vi "UI.vi"() -> ()   [LabVIEW 2016, in "余氯.lvlib"]
uses:
  PLC/PLC.lvlib
  <vilib>/ptbypt/NI_PtbyPt.lvlib
panel:
  in  "测试时间（s）":dbl=60.0
  in  "周期间隔（H）":dbl=4.0
  in  "修正系数":dbl=1.0
  in  "b":dbl=-0.5
  in  "K":dbl=0.000305213
  in  "AD通道":enum16{"AD0", "AD1", "AD2", "AD3", "AD4", "AD5"}(ring)=enum."AD2"
  out "余氯":dbl format="%#.2f"
  # "mg/L"
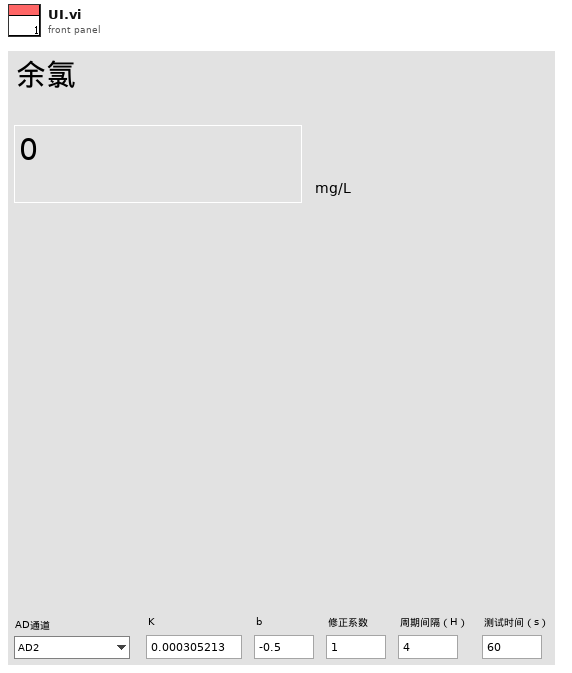
[diagram p1: front panel]
types:
  T1 = cluster{"AD通道":enum16{"AD0", "AD1", "AD2", "AD3", "AD4", "AD5"}, "K":dbl, "b":dbl, "修正系数":dbl, "周期间隔（H）":dbl, "测试时间（s）":dbl}
  T2 = enum16{"空闲", "润洗", "采样", "沉淀", "配水", "反冲洗", "储水", "结束"}
  T3 = typedef "流量计字段定义.ctl" = cluster{"时间":timestamp, "测量模式":string, "数据类型":string, "检测值":sgl, "单位":string, "数据标识":string, "因子编码":string}
  T4 = typedef "LVDateTimeRec.ctl" = cluster{"秒数的小数部分":dbl, "秒":i32, "分":i32, "时":i32, "日":i32, "月":i32, "年":i32, "天数（周）":i32, "天数（年）":i32, "DST":i32}
  T5 = cluster{"AD通道":enum16{"AD0", "AD1", "AD2", "AD3", "AD4", "AD5"}, "K":dbl, "b":dbl, "修正系数":dbl, "数据保存间隔":i32, "测试时间（s）":dbl}
  T6 = cluster{"AD0":i16, "AD1":i16, "AD2":i16, "AD3":i16, "AD4":i16, "AD5":i16}
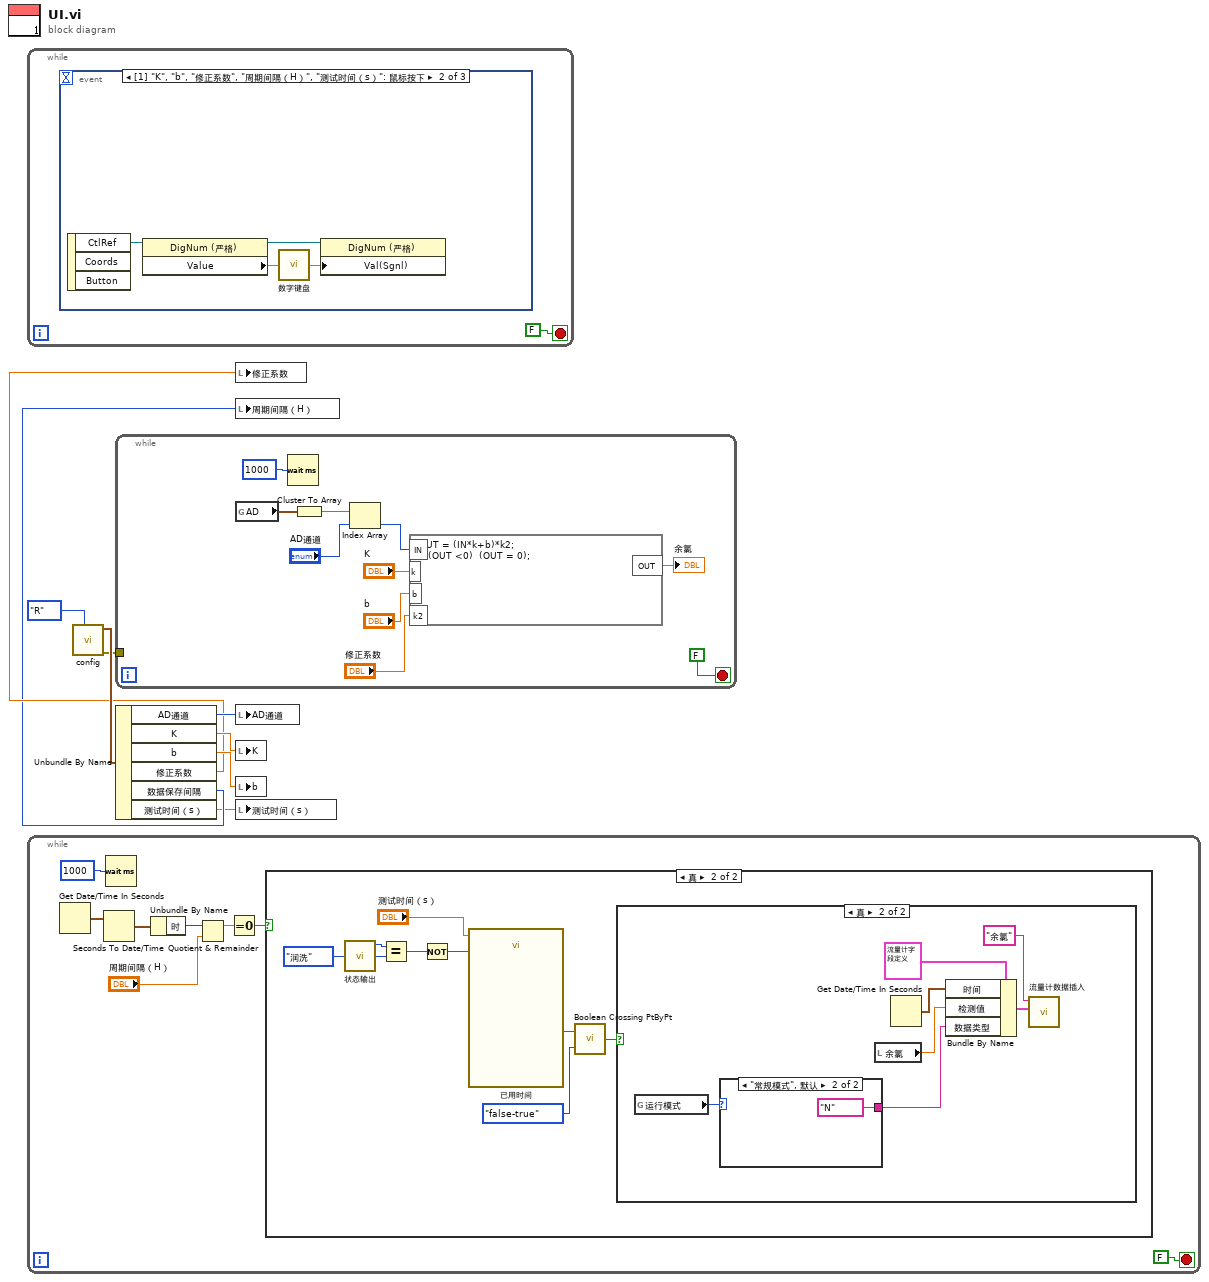
[diagram p0: block diagram]
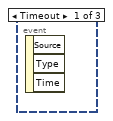
[diagram p2: hidden frame]
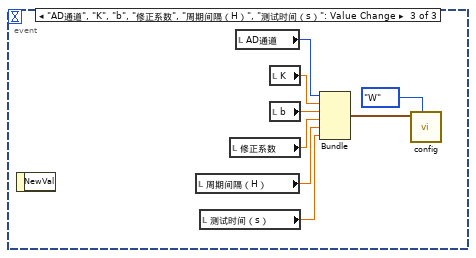
[diagram p3: hidden frame]
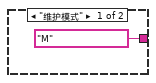
[diagram p6: hidden frame]
diagram:
  n1 = while {
    stop <- FALSE stop-if-true
    n2 = event shown="[1] \"K\", \"b\", \"修正系数\", \"周期间隔（H）\", \"测试时间（s）\": 鼠标按下" {
      selector: _ -> [_ _ _]
      dyn-events: _ -> [_ _ _]
      timeout: _ -> [_ _ _]
      event Timeout {
        n3 = event-data() -> ()  [unwired: 1 in, 3 out]
      }
      event "K", "b", "修正系数", "周期间隔（H）", "测试时间（s）": Mouse Down {
        n4 = event-data() -> ("CtlRef"=w14:refnum<vi>)  [unwired: 1 in, 2 out]
        n5 = property class="DigNum (严格)"(reference=w14) -> (reference out=w12:refnum<vi>, "Value"=w13:dbl)  [unwired: 1 in, 1 out]
        n6 = call "数字键盘.vi"("OldNumber"=w13) -> ("NewNumber"=w11:sgl)
        n7 = property class="DigNum (严格)"(reference=w12, "Val(Sgnl)"=w11) -> ()  [unwired: 1 in, 2 out]
      }
      event "AD通道", "K", "b", "修正系数", "周期间隔（H）", "测试时间（s）": Value Change {
        n8 = event-data() -> ()  [unwired: 1 in, 1 out]
        n9 = local read "周期间隔（H）"() -> (w16:dbl)
        n10 = local read "测试时间（s）"() -> (w15:dbl)
        n11 = local read "修正系数"() -> (w18:dbl)
        n12 = local read "AD通道"() -> (w21:enum16{"AD0", "AD1", "AD2", "AD3", "AD4", "AD5"})
        n13 = local read "K"() -> (w20:dbl)
        n14 = local read "b"() -> (w19:dbl)
        n15 = Bundle("AD通道"=w21, "K"=w20, "b"=w19, "修正系数"=w18, "周期间隔（H）"=w16, "测试时间（s）"=w15) -> (w17:T1)  [unwired: 1 in]
        n16 = call "config.vi"("FUN"=enum16{"R", "W"}."W", "配置输入"=w17) -> ()  [unwired: 8 in, 2 out]
      }
    }
  }
  n17 = while {
    stop <- FALSE stop-if-true
    n18 = Get Date/Time In Seconds() -> (seconds since 1Jan1904=w28:timestamp)
    n19 = Seconds To Date/Time(time stamp (now)=w28) -> (date time rec=w27:T4)  [unwired: 1 in]
    n20 = Wait (ms)(milliseconds to wait=u32 1000 ("等待时间（毫秒）")) -> ()  [unwired: 1 out]
    n21 = Unbundle By Name(w27) -> ("时"=w26:i32)
    n22 = Quotient & Remainder(x=w26, y="周期间隔（H）") -> (x-y*floor(x/y)=w24:dbl)  [unwired: 1 out]
    n23 = Equal To 0?(x=w24) -> (x = 0?=w23:bool)
    n24 = case shown="真" w23 {
      frame False {
      }
      frame True {
        n25 = call "状态输出.vi"() -> ("采配水流程"=w38:T2)  [unwired: 11 in]
        n26 = Equal?(x=w38, y=T2."润洗") -> (x = y?=w33:bool)
        n27 = Not(x=w33) -> (.not. x?=w32:bool)
        n28 = call "已用时间"("Time Target (s)"="测试时间（s）", "Reset"=w32) -> ("Time has Elapsed"=w31:bool)  [unwired: 10 in, 7 out]
        n29 = call <vilib>:"Boolean Crossing PtByPt.vi"("direction"=enum16{"either", "false-true", "true-false"}."false-true", "input"=w31) -> ("crossing"=w36:bool)  [unwired: 1 in]
        n30 = case shown="真" w36 {
          frame False {
          }
          frame True {
            n31 = global read "系统设置全局变量.vi" "运行模式"() -> (w40:enum16{"维护模式", "常规模式", "应急模式", "质控模式"})
            n32 = case shown="\"常规模式\", 默认" w40 {
              tunnel: ["M" ("数据标记表") "N" ("数据标记表")] -> w39
              frame "维护模式" {
              }
              frame "常规模式", Default {
              }
            }
            n33 = local read "余氯"() -> (w42:dbl)
            n34 = Get Date/Time In Seconds() -> (seconds since 1Jan1904=w41:timestamp)
            n35 = Bundle By Name(cluster=T3 {"时间"=timestamp(0 s since 1904-01-01), "测量模式"="水样测试", "数据类型"="N", "检测值"=0.0, "单位"="mg/L", "数据标识"="N", "因子编码"=""} ("data"), "时间"=w41, "检测值"=w42, "数据类型"=w39) -> (w43:T3)
            n36 = call "流量计数据插入.vi"("Tabe Name"="余氯" ("table 输入"), "data"=w43) -> ()  [unwired: 8 in, 1 out]
          }
        }
      }
    }
  }
  n37 = call "config.vi"("FUN"=enum16{"R", "W"}."R") -> ("error out"=w6:errorcluster, "配置输出"=w8:T5)  [unwired: 9 in]
  n38 = while {
    tunnel: w6 -> [_]
    stop <- FALSE stop-if-true
    n39 = global read "采配水全局变量.vi" "AD"() -> (w57:T6)
    n40 = Wait (ms)(milliseconds to wait=u32 1000 ("等待时间（毫秒）")) -> ()  [unwired: 1 out]
    n41 = Cluster To Array(cluster=w57) -> (array=w56:i16[])
    n42 = Index Array(array=w56, index="AD通道") -> (element=w53:i16)
    n43 = formula code="OUT = (IN*k+b)*k2;\nif (OUT <0)  (OUT = 0);"("IN"=w53, "k"="K", "b"="b", "k2"="修正系数") -> ("OUT"=→"余氯":dbl)
  }
  n44 = Unbundle By Name(w8) -> ("AD通道"=w7:enum16{"AD0", "AD1", "AD2", "AD3", "AD4", "AD5"}, "K"=w5:dbl, "b"=w4:dbl, "修正系数"=w3:dbl, "数据保存间隔"=w2:i32, "测试时间（s）"=w1:dbl)
  n45 = local write "修正系数"(w3) -> ()
  n46 = local write "周期间隔（H）"(w2) -> ()
  n47 = local write "AD通道"(w7) -> ()
  n48 = local write "K"(w5) -> ()
  n49 = local write "b"(w4) -> ()
  n50 = local write "测试时间（s）"(w1) -> ()
